vi "Get App Path.vi"() -> (3 "Parent Directory (+ Relative)":path)   [LabVIEW 2025]
uses:
  <userlib>/_OpenG.lib/file/file.llb/openg_file.lvlib
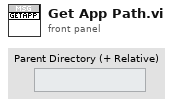
[diagram p1: front panel]
types:
  T1 = enum32{"invalid app kind", "Development System", "Run Time System", "Student Edition", "Embedded LabVIEW", "Evaluation", "Custom"}
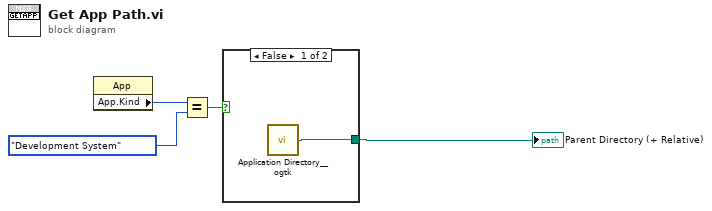
[diagram p0: block diagram]
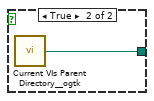
[diagram p2: hidden frame]
diagram:
  n1 = property class="App"() -> ("App.Kind"=w1:T1)  [unwired: 2 in, 2 out]
  n2 = Equal?(x=w1, y=T1."Development System") -> (x = y?=w3:bool)
  n3 = case shown="False" w3 {
    tunnel: [w5 w6] -> w4
    frame False {
      n4 = call <userlib>:"Application Directory__ogtk.vi"() -> ("Application Directory (+ Relative)"=w5:path)  [unwired: 1 in]
    }
    frame True {
      n5 = call <userlib>:"Current VIs Parent Directory__ogtk.vi"() -> ("Parent Directory (+ Relative)"=w6:path)  [unwired: 5 in]
    }
  }
  "Parent Directory (+ Relative)" <- w4
